vi "WillDey_SetPowerSupply.vi"() -> ()   [LabVIEW 2017]
uses:
  Globals/WillDey_Channels.vi
panel:
  in  "Voltage":dbl
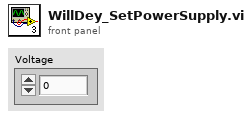
[diagram p1: front panel]
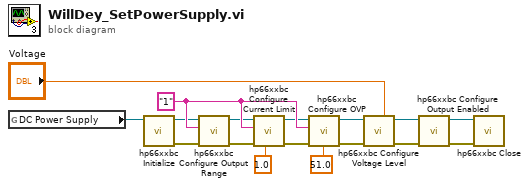
[diagram p0: block diagram]
diagram:
  w13 = "1" ("channel (\"\") name")
  n1 = global read "WillDey_Channels.vi" "DC Power Supply"() -> (w4:refnum<k15>)
  n2 = call <instrlib>:"hp66xxbc Initialize.vi"("resource name (\"GPIB::14::INSTR\")"=w4) -> ("error out"=w8:errorcluster, "instrument handle"=w9:refnum<k15>)  [unwired: 9 in]
  n3 = call <instrlib>:"hp66xxbc Configure Output Range.vi"("error in (no error)"=w8, "channel name (\"\")"=w13, "instrument handle"=w9) -> ("error out"=w5:errorcluster, "instrument handle out"=w6:refnum<k15>)  [unwired: 7 in]
  n4 = call <instrlib>:"hp66xxbc Configure Current Limit.vi"("limit (0.00 A)"=1.0, "error in (no error)"=w5, "channel name (\"\")"=w13, "instrument handle"=w6) -> ("error out"=w10:errorcluster, "instrument handle out"=w11:refnum<k15>)  [unwired: 6 in]
  n5 = call <instrlib>:"hp66xxbc Configure OVP.vi"("limit (0.0 V)"=51.0, "error in (no error)"=w10, "channel name (\"\")"=w13, "instrument handle"=w11) -> ("error out"=w17:errorcluster, "instrument handle out"=w16:refnum<k15>)  [unwired: 6 in]
  n6 = call <instrlib>:"hp66xxbc Configure Voltage Level.vi"("error in (no error)"=w17, "level (0.0)"="Voltage", "instrument handle"=w16) -> ("error out"=w14:errorcluster, "instrument handle out"=w15:refnum<k15>)  [unwired: 7 in]
  n7 = call <instrlib>:"hp66xxbc Configure Output Enabled.vi"("error in (no error)"=w14, "instrument handle"=w15) -> ("error out"=w2:errorcluster, "instrument handle out"=w1:refnum<k15>)  [unwired: 8 in]
  n8 = call <instrlib>:"hp66xxbc Close.vi"("error in (no error)"=w2, "instrument handle"=w1) -> ()  [unwired: 9 in, 1 out]
